vi "Watlow Loop.vi"() -> ()   [LabVIEW 2013]
uses:
  Modbus Mode.ctl
  Type Defs/Pump Data Mode.ctl
panel:
  out "Watlow Present":bool
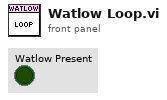
[diagram p1: front panel]
types:
  T1 = typedef "Modbus Mode.ctl" = enum16{"Init", "Tank 1 Write", "Tank 2 Write", "Tank 1 Read", "Tank 2 Read"}
  T2 = typedef "Pump Data Mode.ctl" = enum16{"Read", "Write Data", "Write Cal", "Write Watlow Data", "Write Pressure Offsets", "Write Initial Times", "Write Pumps Present", "Diagnostic Status", "Write Speed"}
  T3 = typedef "Tank Temp Variables.ctl" = cluster{"Tank 1 Temp":sgl, "Tank 1 Setpoint":sgl, "Tank 2 Temp":sgl, "Tank 2 Setpoint":sgl}
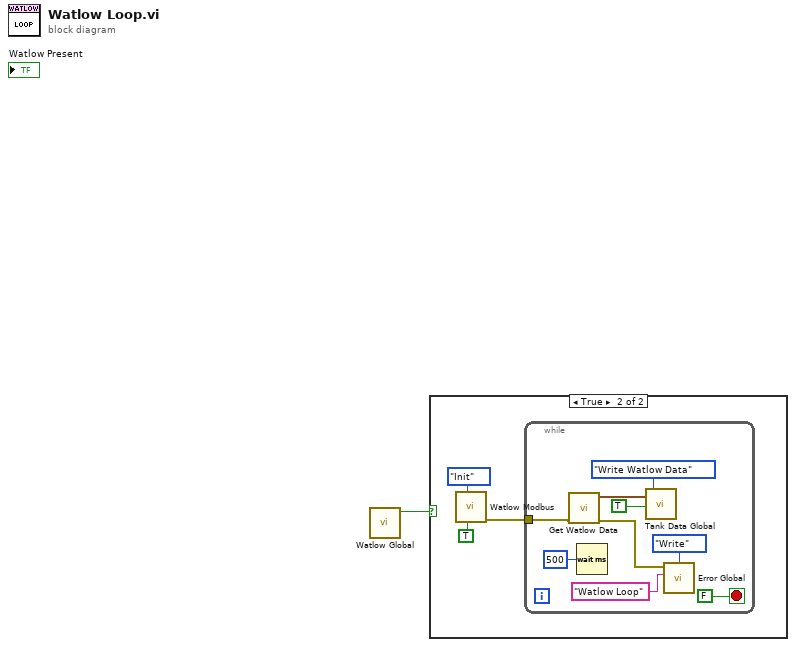
[diagram p0: block diagram]
diagram:
  n1 = call "Watlow Global.vi"() -> ("Watlow Present OUT"=w1:bool)  [unwired: 11 in]
  n2 = case shown="True" w1 {
    frame False {
    }
    frame True {
      n3 = call "Watlow Modbus.vi"("Watlow Present?"=TRUE, "Modbus Mode"=Modbus_Mode."Init") -> ("Error OUT"=w3:errorcluster)  [unwired: 8 in, 1 out]
      n4 = while {
        tunnel: w3 -> [w8]
        stop <- FALSE stop-if-true
        n5 = call "Get Watlow Data.vi"("Error IN"=w8) -> ("Error OUT"=w7:errorcluster, "Tank Temp Variables"=w10:T3)  [unwired: 8 in, 1 out]
        n6 = Wait (ms)(milliseconds to wait=u32 500) -> ()  [unwired: 1 out]
        n7 = call "Tank Data Global.vi"("Tank Temp Variables"=w10, "Watlow Present"=TRUE, "Pump Data Mode"=Pump_Data_Mode."Write Watlow Data") -> ()  [unwired: 11 in, 6 out]
        n8 = call "Error Global.vi"("Mode"=enum16{"Read", "Write", "Clear Error"}."Write", "Error In"=w7, "Location In"="Watlow Loop") -> ()  [unwired: 6 in, 2 out]
      }
    }
  }
